vi "LinearSystemSim_SetInput_Array.vi"(9 "Input":dbl[](array[numeric]), 11 "in LinearSystemSim":T1) -> (0 "Size Coerced":bool, 3 "out LinearSystemSim":T1)   [LabVIEW 2019, in "Trajectory_Library.lvlib"]
doc: "Sets the system inputs.\n \nInputs:\n - LinearSystemSim -- Data cluster\n - Inputs -- An array of doubles that represent the inputs (u) of the system.\n\nOutputs:\n - OutLinearSystemSim -- Updated data cluster\n - SizeCoerced -- If TRUE, an error occured. Execution may continue."
uses:
  Trajectory_Library.lvlib
  LINEAR_SYSTEM_SIM.ctl
  LINEAR_SYSTEM.ctl
  <vilib>/Analysis/Matrix/Datatypes/RealMatrix.ctl
  MatBuilder_Create.vi
  <vilib>/Analysis/Matrix/NI_Matrix.lvlib
panel:
  # "<States, 1>"
  # "<Outputs, 1>"
  # "<Inputs, 1>"
  # "<Outputs, 1>"
  # "<States,States>"
  # "<States,Inputs>"
  # "<Outputs,States>"
  # "<Outputs,Inputs>"
  # "<States, 1>"
  # "<Outputs, 1>"
  # "<Inputs, 1>"
  # "<Outputs, 1>"
  # "<States,States>"
  # "<States,Inputs>"
  # "<Outputs,States>"
  # "<Outputs,Inputs>"
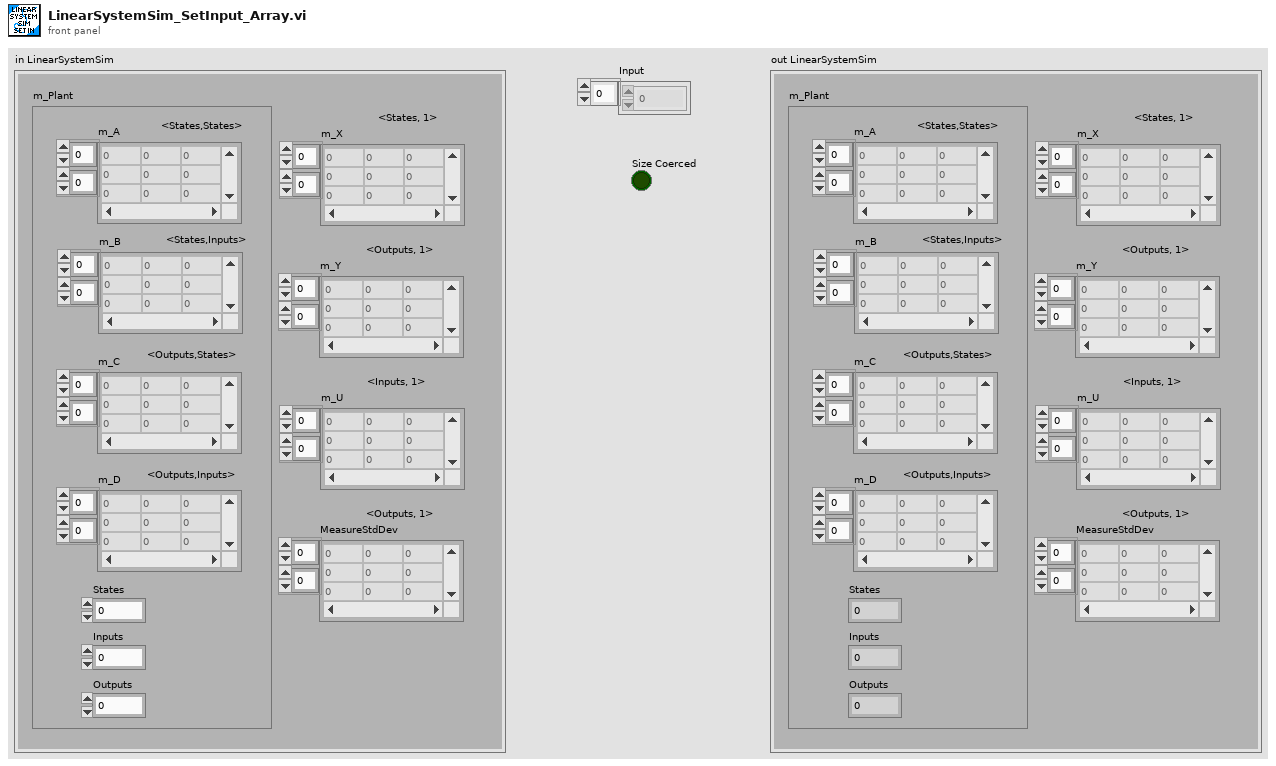
[diagram p1: front panel]
types:
  T1 = typedef "Trajectory_Library.lvlib/LINEAR_SYSTEM_SIM.ctl" = cluster{"m_Plant":T2, "m_X":T3, "m_Y":T3, "m_U":T3, "MeasureStdDev":T3}
  T2 = typedef "Trajectory_Library.lvlib/LINEAR_SYSTEM.ctl" = cluster{"m_A":T3, "m_B":T3, "m_C":T3, "m_D":T3, "States":i32, "Inputs":i32, "Outputs":i32}
  T3 = typedef "NI_Matrix.lvlib/RealMatrix.ctl" = dbl[][]
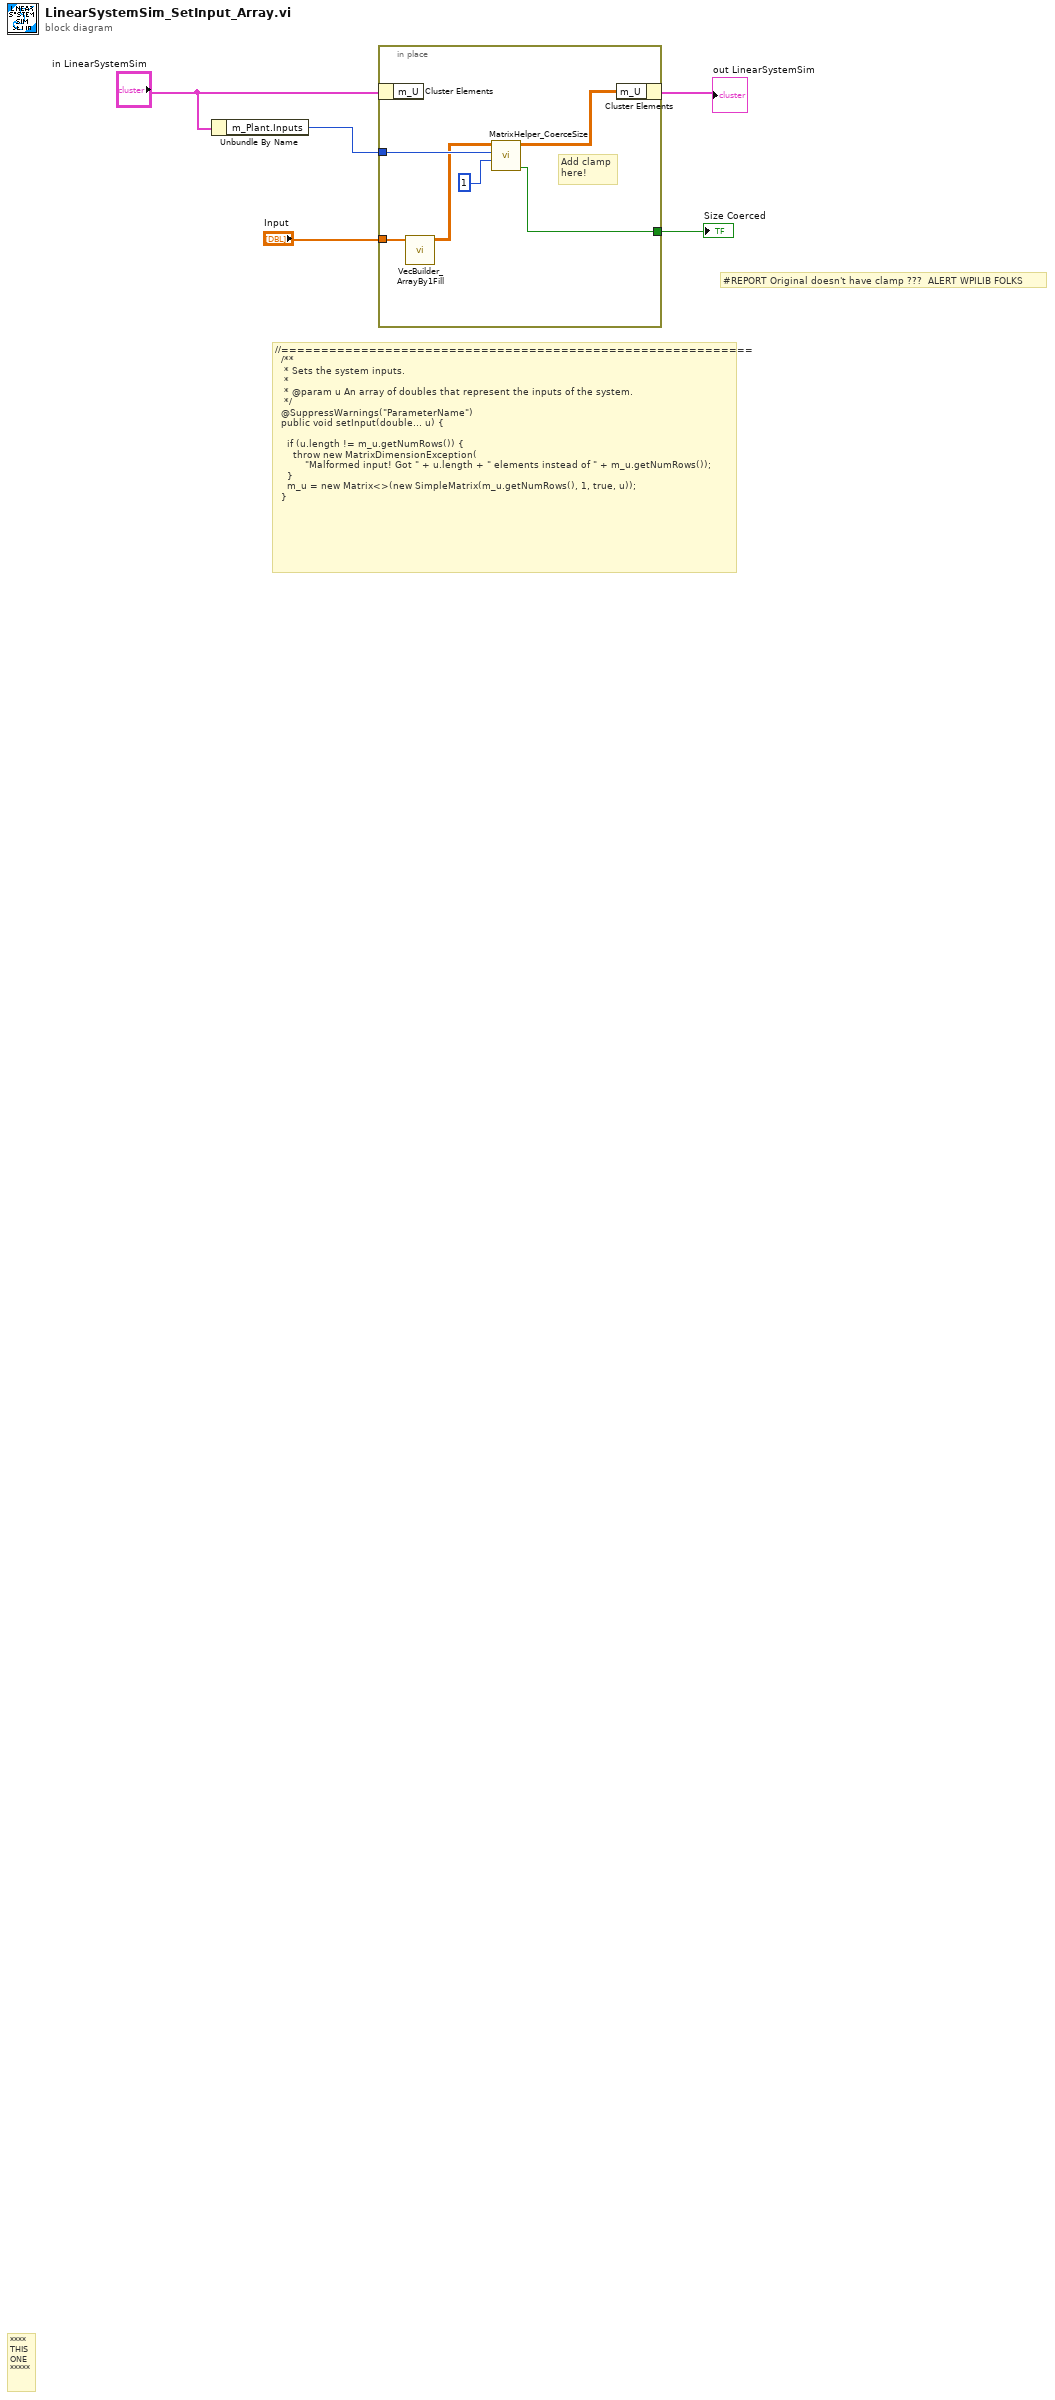
[diagram p0: block diagram]
diagram:
  # "#REPORT Original doesn't have clamp ???  ALERT WPILIB FOLKS"
  # "//===========================================================\n  /**\n   * Sets the system inputs.\n   *\n   * @param u An array of doubles that represent the inputs of the system.\n   */\n  @SuppressWarnings(\"ParameterName\")\n  public void setInput(double... u) {\n\n    if (u.length != m_u.getNumRows()) {\n      throw new MatrixDimensionException(\n          \"Malformed input! Got \" + u.length + \" elements instead of \" + m_u.getNumRows());\n    }\n    m_u = new Matrix<>(new SimpleMatrix(m_u.getNumRows(), 1, true, u));\n  }"
  # "****\nTHIS\nONE\n*****"
  n1 = Unbundle By Name("in LinearSystemSim") -> ("m_Plant.Inputs"=w2:i32)
  n2 = in-place {
    in-place-border: "Input" -> [w8]
    in-place-border: w2 -> [w10]
    in-place-border: [w6] -> w1
    # "Add clamp\nhere!"
    n3 = in-place-cluster #1("in LinearSystemSim") -> ()  [unwired: 1 out]
    n4 = call "VecBuilder_ArrayBy1Fill.vi"("R Array"=w8) -> ("Output Vector"=w7:T3)  [unwired: 10 in]
    n5 = call "MatrixHelper_CoerceSize.vi"("Columns"=1, "Rows"=w10, "input matrix"=w7) -> ("Coerced"=w6:bool, "output matrix"=w9:T3)  [unwired: 7 in]
    n6 = in-place-cluster #1("m_U"=w9) -> (→"out LinearSystemSim":T1)
  }
  "Size Coerced" <- w1
